vi "Initialize.vi"(8 "error in (no error)":errorcluster, 11 "WebSocket Client in":refnum<class "WebSocket Client.lvclass">) -> (0 "error out":errorcluster, 3 "WebSocket Client out":refnum<class "WebSocket Client.lvclass">)   [LabVIEW 2021, in "WebSockets.lvlib" / "WebSocket Client.lvclass"]
doc: "Opens a conenction and creates a new WebSocket Client using the NI VISA TCP Socket.\nWebSockets 2.0.1.40\nSam Sharp - MediaMongrels Ltd\nCopyright (c) 2019, MediaMongrels Ltd"
uses:
  WebSocket Client.lvclass
  WebSocket Client.lvclass/WebSocket Client.ctl
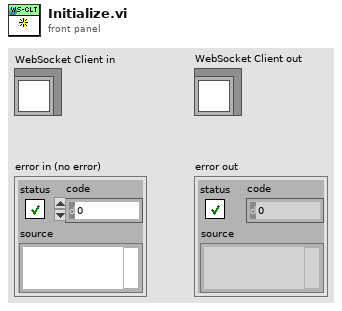
[diagram p1: front panel]
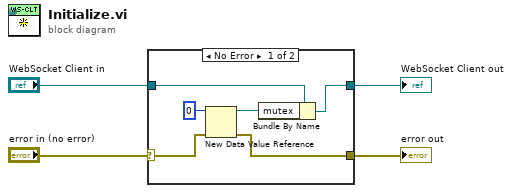
[diagram p0: block diagram]
diagram:
  n1 = case shown="No Error" "error in (no error)" {
    selector: "error in (no error)" -> [w6 w12]
    tunnel: "WebSocket Client in" -> [w9 w11]
    tunnel: [w8 w11] -> w1
    tunnel: [w7 w12] -> w3
    frame No Error {
      n2 = New Data Value Reference(data value=u8 0, error in=w6) -> (data value reference=w5:refnum<data-value>, error out=w7:errorcluster)
      n3 = Bundle By Name(cluster=w9, "mutex"=w5) -> (w8:refnum<class "WebSocket Client.lvclass">)
    }
    frame Error {
    }
  }
  "error out" <- w3
  "WebSocket Client out" <- w1
